vi "LINC Session Global.vi"(5 "target name":string, 6 "value in":i32, 7 "mode":T2, 8 "error in (no error)":errorcluster, 9 "reference in":refnum<vi>, 10 "listener in":refnum<k5>, 11 "connection in":refnum<k5>) -> (0 "error out":errorcluster, 1 "reference out":refnum<vi>[](array[refnum]), 2 "listener out":refnum<k5>[](array[refnum]), 3 "connections out":refnum<k5>[](array[refnum]), 4 "port config":T1[](array[typedef]))   [LabVIEW 2018, in "STEPkgDriver_LINC.lvlib"]
uses:
  STEPkgDriver_LINC.lvlib
  LINC Port Config.ctl
  LINC.lvclass
  LINC Global Session Mode.ctl
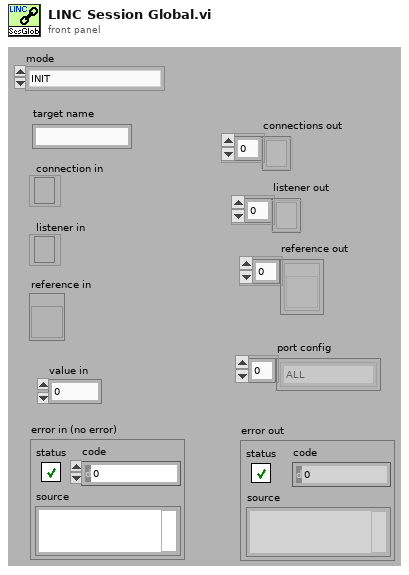
[diagram p1: front panel]
types:
  T1 = typedef "STEPkgDriver_LINC.lvlib/LINC Port Config.ctl" = enum16{"ALL", "CMD_ALL", "TLM_ALL", "TLM_BASIC"}
  T2 = typedef "STEPkgDriver_LINC.lvlib/LINC Global Session Mode.ctl" = enum16{"INIT", "CLEAR", "ADD_SESSION", "SET_CONNECTION", "SET_LISTENER", "SET_REFERENCE", "GET_SESSION"}
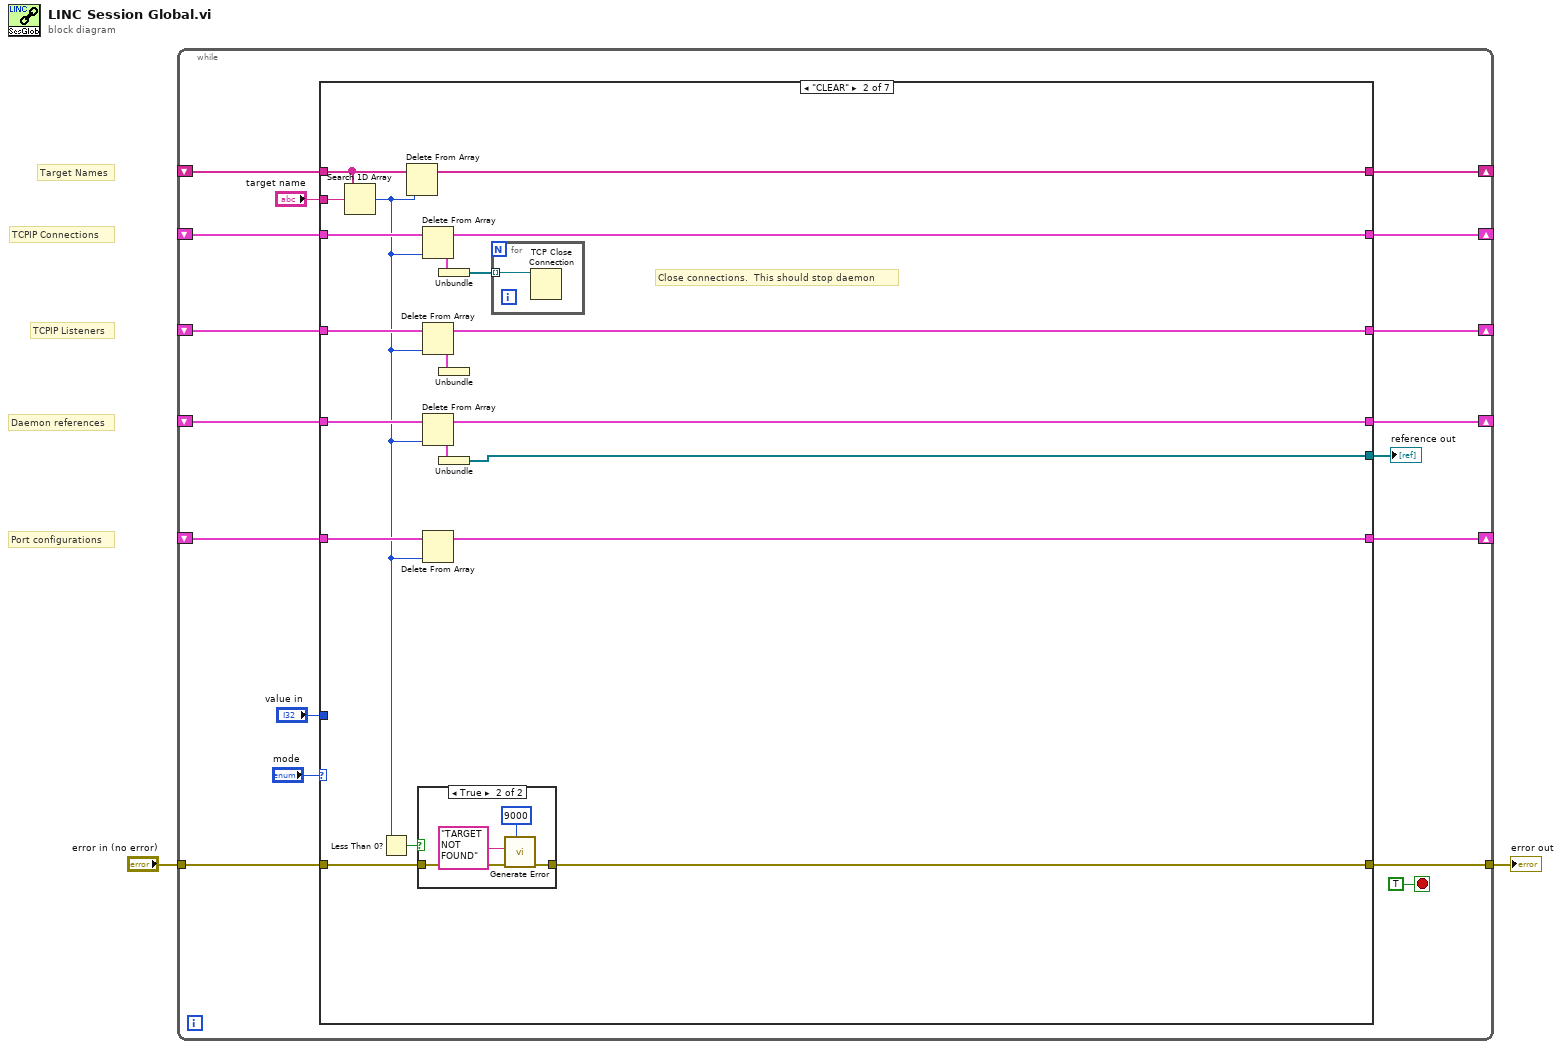
[diagram p0: block diagram]
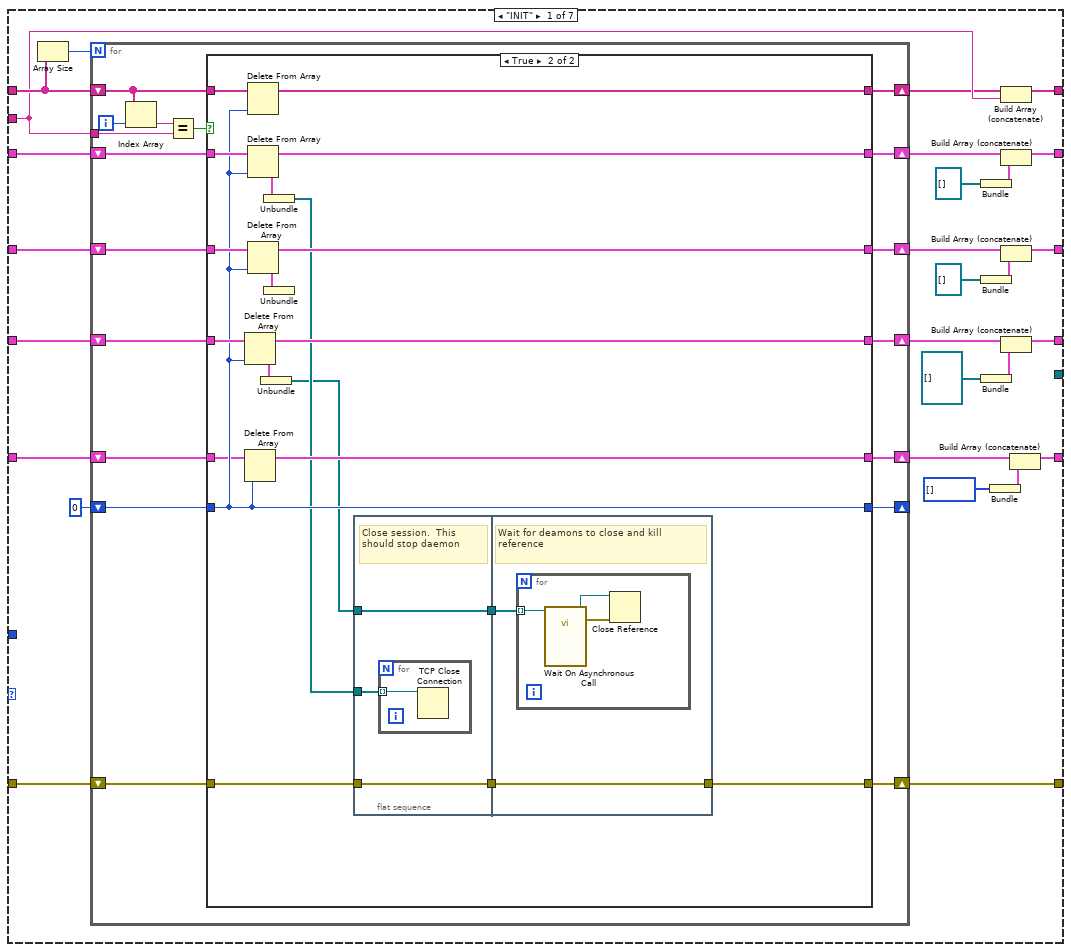
[diagram p2: hidden frame]
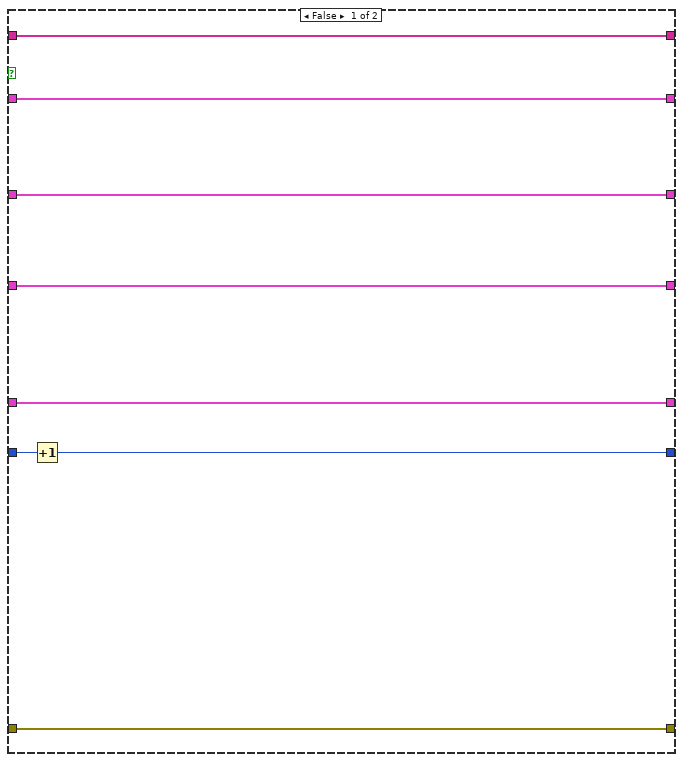
[diagram p3: hidden frame]
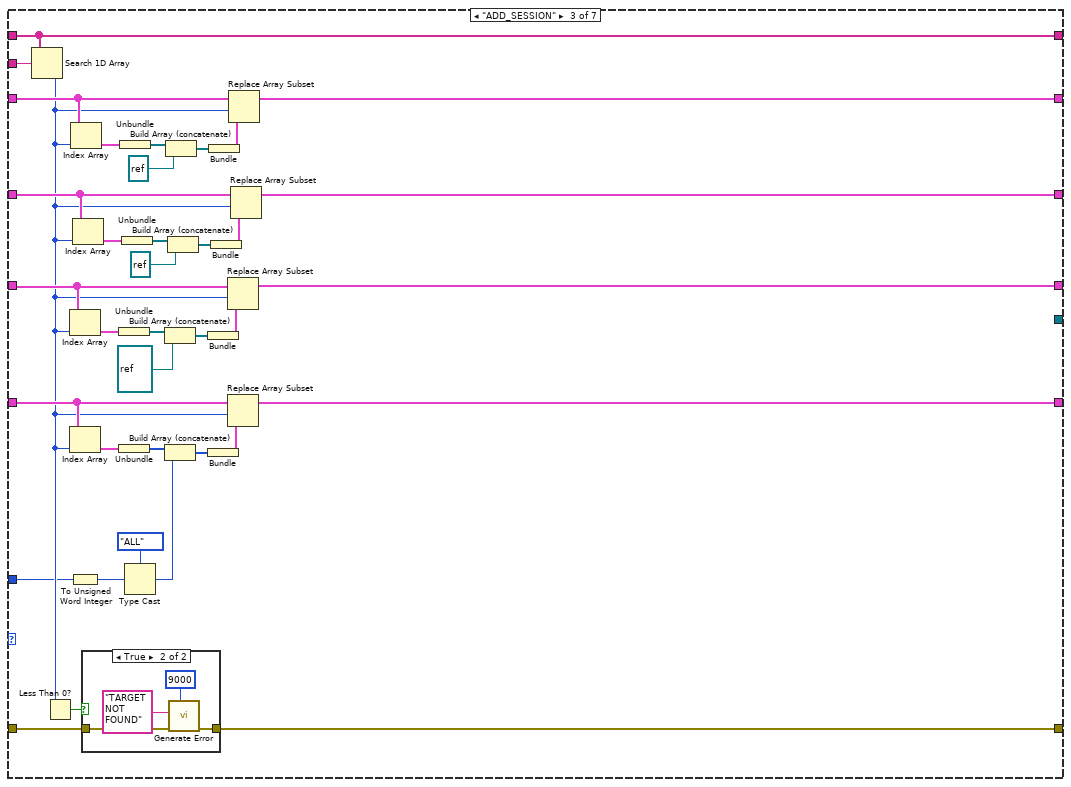
[diagram p5: hidden frame]
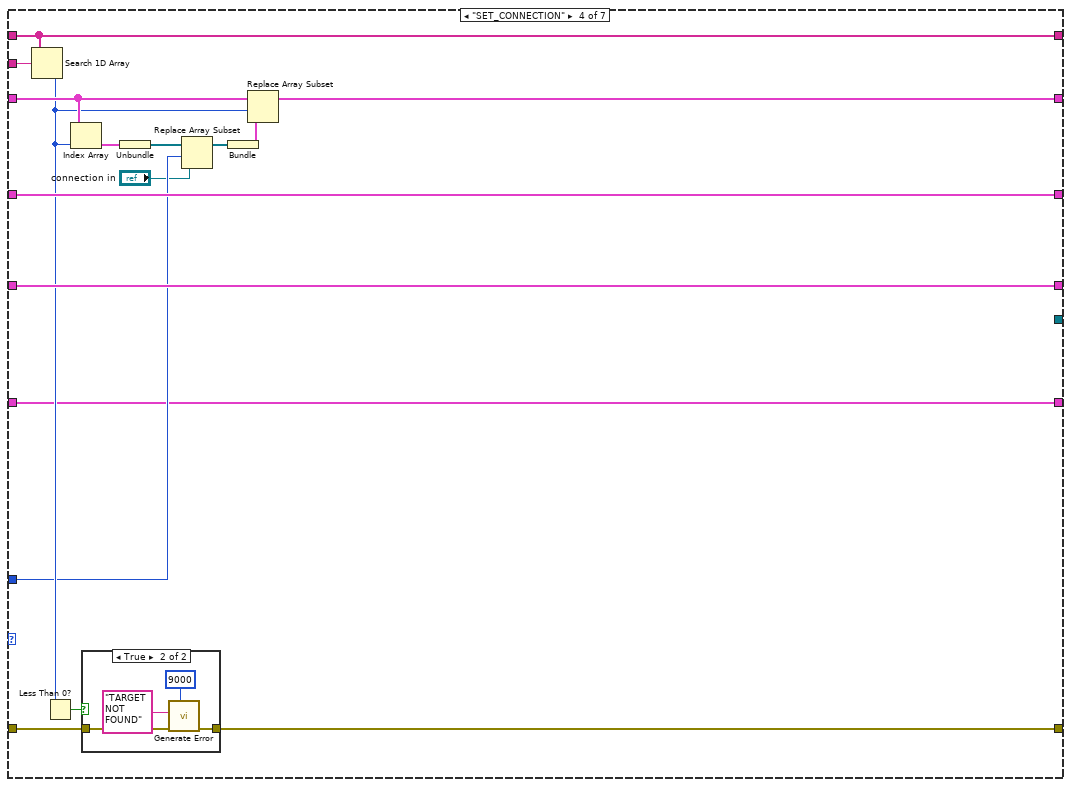
[diagram p7: hidden frame]
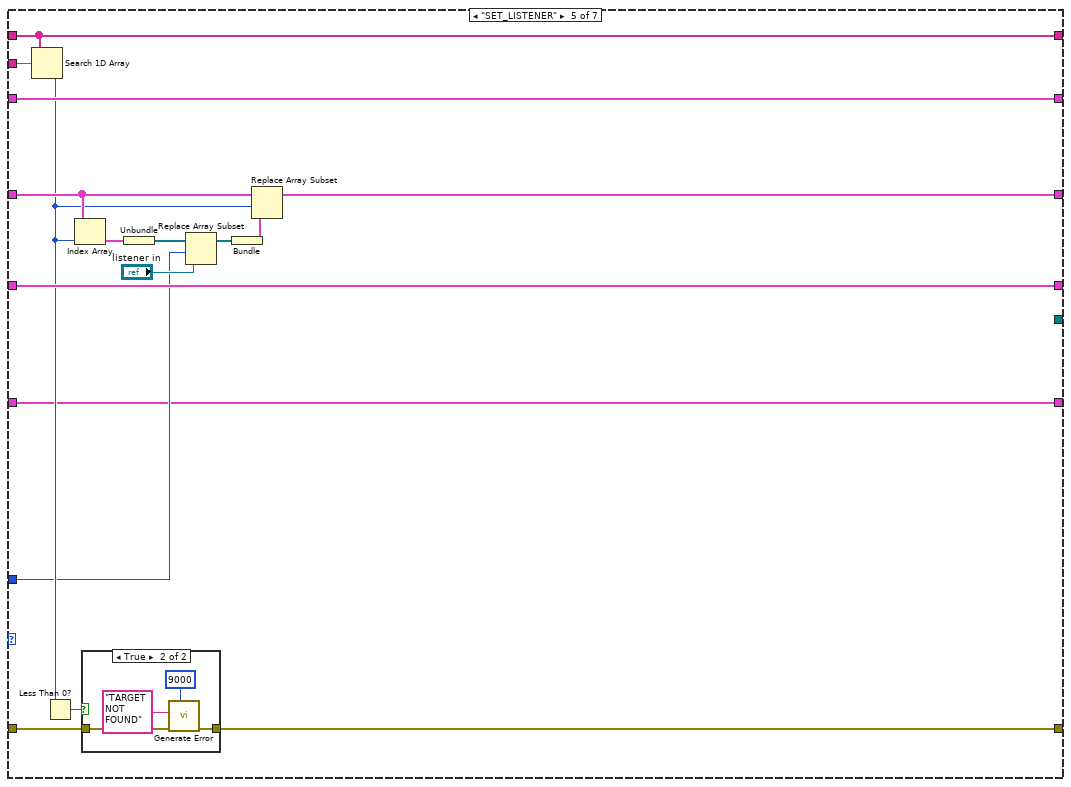
[diagram p9: hidden frame]
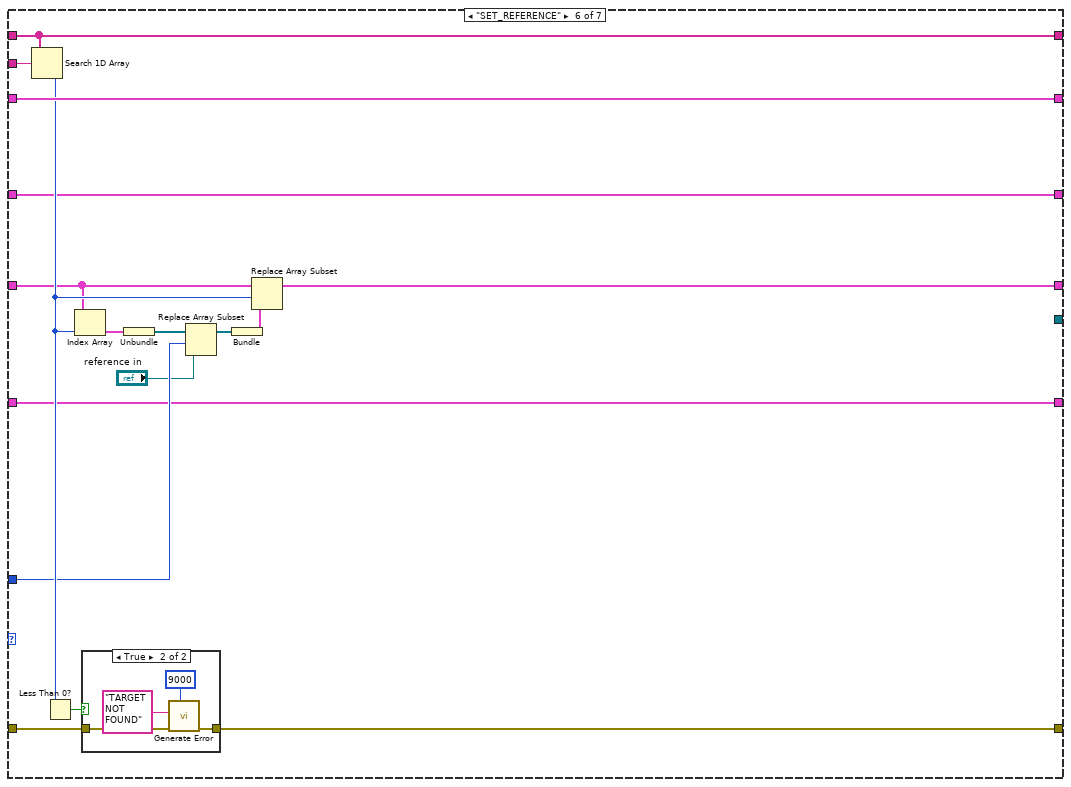
[diagram p11: hidden frame]
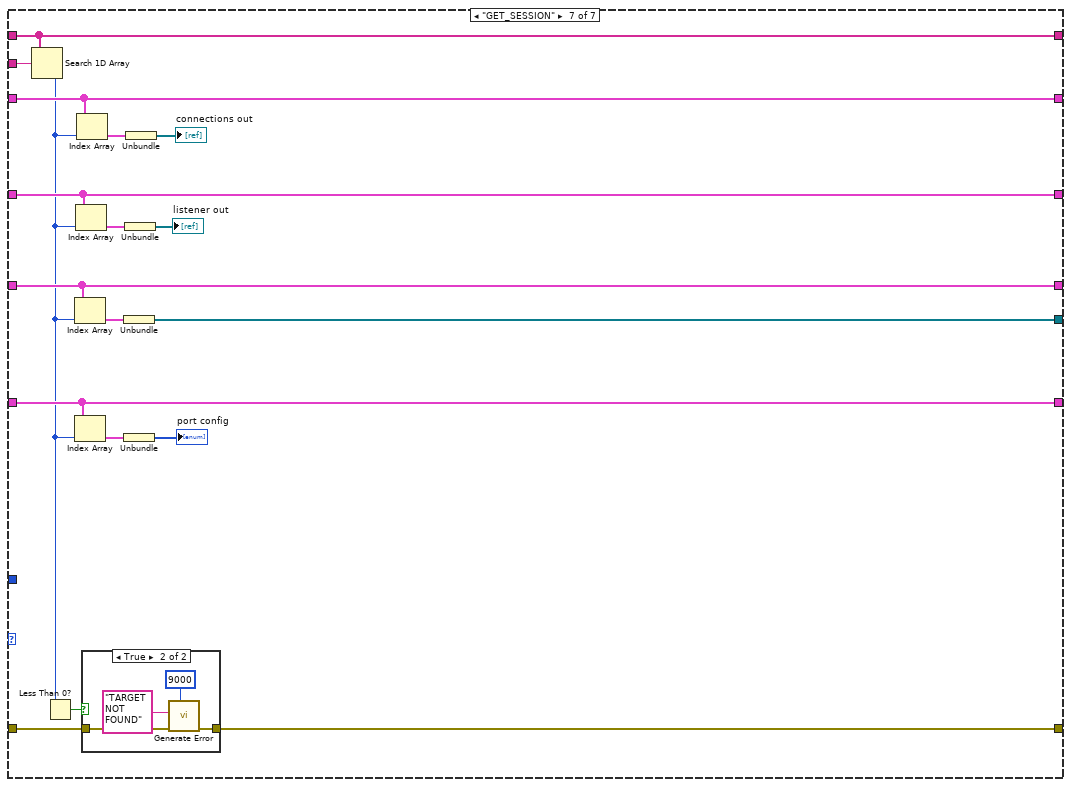
[diagram p13: hidden frame]
diagram:
  # "Target Names"
  # "Port configurations"
  # "Daemon references"
  # "TCPIP Listeners"
  # "TCPIP Connections"
  n1 = while {
    shift-right: [w17] -> _
    shift-left: _ -> [w18]
    tunnel: "error in (no error)" -> [w14]
    tunnel: [w13] -> w1
    shift-right: [w11] -> _
    shift-left: _ -> [w12]
    shift-right: [w9] -> _
    shift-left: _ -> [w10]
    shift-right: [w8] -> _
    shift-left: _ -> [w7]
    shift-right: [w4] -> _
    shift-left: _ -> [w5]
    stop <- TRUE stop-if-true
    n2 = case shown="\"CLEAR\"" "mode" {
      tunnel: w18 -> [w36 w121 w164 w186 w208 w230 w253]
      tunnel: [w47 w120 w164 w186 w208 w230 w253] -> w17
      tunnel: "target name" -> [w34 w122 w165 w187 w209 w231 w254]
      tunnel: w14 -> [w21 w118 w160 w183 w205 w227 w251]
      tunnel: [w20 w104 w161 w182 w204 w226 w250] -> w13
      tunnel: w12 -> [w33 w117 w159 w178 w207 w229 w249]
      tunnel: [w46 w116 w163 w177 w207 w229 w249] -> w11
      tunnel: w10 -> [w30 w115 w148 w185 w198 w218 w245]
      tunnel: [w41 w114 w147 w185 w197 w218 w245] -> w9
      tunnel: w7 -> [w29 w113 w142 w181 w203 w219 w244]
      tunnel: [w40 w112 w141 w181 w203 w217 w244] -> w8
      tunnel: "value in" -> [_ _ w133 w173 w194 w220 _]
      tunnel: w5 -> [w25 w108 w136 w171 w193 w216 w240]
      tunnel: [w23 w107 w135 w171 w193 w216 w240] -> w4
      tunnel: [_ w103 _ _ _ _ w237] -> w3
      frame "INIT" {
        w26 = T1[] [] items=["ALL", "CMD_ALL", "TLM_ALL", "TLM_BASIC"]
        n3 = Array Size(array=w36) -> (size(s)=w35:i32)
        n4 = for {
          N: w35 -> [_]
          shift-right: [w58] -> w32
          shift-left: w36 -> [w64]
          shift-right: [w57] -> w31
          shift-left: w33 -> [w63]
          shift-right: [w56] -> w28
          shift-left: w30 -> [w62]
          tunnel: w34 -> [w60]
          shift-right: [w54] -> _
          shift-left: 0 -> [w55]
          shift-right: [w53] -> w27
          shift-left: w29 -> [w52]
          shift-right: [w50] -> w24
          shift-left: w25 -> [w51]
          shift-right: [w48] -> w20
          shift-left: w21 -> [w49]
          i -> [w65]
          n5 = Index Array(array=w64, index=w65) -> (element=w61:string)
          n6 = Equal?(x=w61, y=w60) -> (x = y?=w59:bool)
          n7 = case shown="True" w59 {
            tunnel: w64 -> [w73 w93]
            tunnel: w63 -> [w72 w91]
            tunnel: w62 -> [w71 w90]
            tunnel: [w73 w92] -> w58
            tunnel: [w72 w89] -> w57
            tunnel: [w71 w88] -> w56
            tunnel: w55 -> [w70 w82]
            tunnel: [w69 w82] -> w54
            tunnel: w52 -> [w68 w86]
            tunnel: [w68 w87] -> w53
            tunnel: w51 -> [w67 w81]
            tunnel: [w67 w80] -> w50
            tunnel: w49 -> [w66 w79]
            tunnel: [w66 w78] -> w48
            frame False {
              n8 = Increment(x=w70) -> (x+1=w69:i32)
            }
            frame True {
              n9 = Delete From Array(array=w86, index=w82) -> (deleted portion=w83:cluster{refnum<vi>[]}, array with subset deleted=w87:cluster{refnum<vi>[]}[])  [unwired: 1 in]
              n10 = Delete From Array(array=w81, index=w82) -> (array with subset deleted=w80:cluster{T1[]}[])  [unwired: 1 in, 1 out]
              n11 = Delete From Array(array=w93, index=w82) -> (array with subset deleted=w92:string[])  [unwired: 1 in, 1 out]
              n12 = Delete From Array(array=w91, index=w82) -> (deleted portion=w85:cluster{refnum<k5>[]}, array with subset deleted=w89:cluster{refnum<k5>[]}[])  [unwired: 1 in]
              n13 = Delete From Array(array=w90, index=w82) -> (deleted portion=w84:cluster{refnum<k5>[]}, array with subset deleted=w88:cluster{refnum<k5>[]}[])  [unwired: 1 in]
              n14 = Unbundle(w83) -> (w76:refnum<vi>[])
              n15 = Unbundle(w85) -> (w77:refnum<k5>[])
              n16 = Unbundle(w84) -> ()  [unwired: 1 out]
              n17 = flat-sequence {
                tunnel: w79 -> [w96]
                tunnel: [w96] -> w75
                tunnel: w77 -> [w95]
                tunnel: [w94] -> w74
                tunnel: w76 -> [w94]
                tunnel: w75 -> [w98]
                tunnel: w74 -> [w99]
                tunnel: [w98] -> w78
                frame #0 {
                  # "Close session.  This should stop daemon"
                  n18 = for {
                    tunnel: w95 -> [w97] mode=indexing
                    n19 = TCP Close Connection(connection ID=w97) -> ()  [unwired: 2 in, 2 out]
                  }
                }
                frame #1 {
                  # "Wait for deamons to close and kill reference"
                  n20 = for {
                    tunnel: w99 -> [w102] mode=indexing
                    n21 = call-by-ref "Wait On Asynchronous Call"(reference=w102) -> (reference out=w100:refnum<vi>, error out=w101:errorcluster)  [unwired: 13 in]
                    n22 = Close Reference(reference=w100, error in (no error)=w101) -> ()  [unwired: 1 out]
                  }
                }
              }
            }
          }
        }
        n23 = Bundle(refnum<k5>[] []) -> (w44:cluster{refnum<k5>[]})  [unwired: 1 in]
        n24 = Bundle(refnum<k5>[] []) -> (w43:cluster{refnum<k5>[]})  [unwired: 1 in]
        n25 = Bundle(refnum<vi>[] []) -> (w38:cluster{refnum<vi>[]})  [unwired: 1 in]
        n26 = Bundle(w26) -> (w22:cluster{T1[]})  [unwired: 1 in]
        n27 = Build Array (concatenate)(w32, w34) -> (w47:string[])
        n28 = Build Array (concatenate)(w31, w44) -> (w46:cluster{refnum<k5>[]}[])
        n29 = Build Array (concatenate)(w28, w43) -> (w41:cluster{refnum<k5>[]}[])
        n30 = Build Array (concatenate)(w27, w38) -> (w40:cluster{refnum<vi>[]}[])
        n31 = Build Array (concatenate)(w24, w22) -> (w23:cluster{T1[]}[])
      }
      frame "CLEAR" {
        # "Close connections.  This should stop daemon"
        n32 = Search 1D Array(1D array=w121, element=w122) -> (index of element=w106:i32)  [unwired: 1 in]
        n33 = Less Than 0?(x=w106) -> (x < 0?=w119:bool)
        n34 = Delete From Array(array=w121, index=w106) -> (array with subset deleted=w120:string[])  [unwired: 1 in, 1 out]
        n35 = case shown="True" w119 {
          tunnel: w118 -> [w124 w128]
          tunnel: [w124 w127] -> w104
          frame False {
          }
          frame True {
            n36 = call "Generate Error.vi"("error code (-1301)"=9000, "error in"=w128, "description"="TARGET NOT FOUND") -> ("error out"=w127:errorcluster)  [unwired: 8 in]
          }
        }
        n37 = Delete From Array(array=w117, index=w106) -> (deleted portion=w111:cluster{refnum<k5>[]}, array with subset deleted=w116:cluster{refnum<k5>[]}[])  [unwired: 1 in]
        n38 = Delete From Array(array=w115, index=w106) -> (deleted portion=w110:cluster{refnum<k5>[]}, array with subset deleted=w114:cluster{refnum<k5>[]}[])  [unwired: 1 in]
        n39 = Delete From Array(array=w113, index=w106) -> (deleted portion=w109:cluster{refnum<vi>[]}, array with subset deleted=w112:cluster{refnum<vi>[]}[])  [unwired: 1 in]
        n40 = Delete From Array(array=w108, index=w106) -> (array with subset deleted=w107:cluster{T1[]}[])  [unwired: 1 in, 1 out]
        n41 = Unbundle(w111) -> (w105:refnum<k5>[])
        n42 = Unbundle(w110) -> ()  [unwired: 1 out]
        n43 = Unbundle(w109) -> (w103:refnum<vi>[])
        n44 = for {
          tunnel: w105 -> [w123] mode=indexing
          n45 = TCP Close Connection(connection ID=w123) -> ()  [unwired: 2 in, 2 out]
        }
      }
      frame "ADD_SESSION" {
        n46 = Search 1D Array(1D array=w164, element=w165) -> (index of element=w134:i32)  [unwired: 1 in]
        n47 = Less Than 0?(x=w134) -> (x < 0?=w162:bool)
        n48 = Index Array(array=w142, index=w134) -> (element=w146:cluster{refnum<vi>[]})
        n49 = Index Array(array=w136, index=w134) -> (element=w137:cluster{T1[]})
        n50 = To Unsigned Word Integer(number=w133) -> (unsigned 16bit integer=w130:u16)
        n51 = Index Array(array=w159, index=w134) -> (element=w158:cluster{refnum<k5>[]})
        n52 = Index Array(array=w148, index=w134) -> (element=w149:cluster{refnum<k5>[]})
        n53 = case shown="True" w162 {
          tunnel: w160 -> [w166 w170]
          tunnel: [w166 w169] -> w161
          frame False {
          }
          frame True {
            n54 = call "Generate Error.vi"("error code (-1301)"=9000, "error in"=w170, "description"="TARGET NOT FOUND") -> ("error out"=w169:errorcluster)  [unwired: 8 in]
          }
        }
        n55 = Unbundle(w146) -> (w145:refnum<vi>[])
        n56 = Unbundle(w137) -> (w138:T1[])
        n57 = Unbundle(w158) -> (w157:refnum<k5>[])
        n58 = Unbundle(w149) -> (w150:refnum<k5>[])
        n59 = Type Cast(type=LINC_Port_Config."ALL" ("port config"), x=w130) -> (*(type *) &x=w131:T1)
        n60 = Build Array (concatenate)(w145, refnum<vi> refnum) -> (w144:refnum<vi>[])
        n61 = Build Array (concatenate)(w138, w131) -> (w139:T1[])
        n62 = Build Array (concatenate)(w157, refnum<k5> refnum ("connection in")) -> (w155:refnum<k5>[])
        n63 = Build Array (concatenate)(w150, refnum<k5> refnum ("connection in")) -> (w152:refnum<k5>[])
        n64 = Bundle(w144) -> (w143:cluster{refnum<vi>[]})  [unwired: 1 in]
        n65 = Bundle(w139) -> (w140:cluster{T1[]})  [unwired: 1 in]
        n66 = Bundle(w155) -> (w154:cluster{refnum<k5>[]})  [unwired: 1 in]
        n67 = Bundle(w152) -> (w153:cluster{refnum<k5>[]})  [unwired: 1 in]
        n68 = Replace Array Subset(array=w142, new element=w143, index=w134) -> (w141:cluster{refnum<vi>[]}[])
        n69 = Replace Array Subset(array=w136, new element=w140, index=w134) -> (w135:cluster{T1[]}[])
        n70 = Replace Array Subset(array=w159, new element=w154, index=w134) -> (w163:cluster{refnum<k5>[]}[])
        n71 = Replace Array Subset(array=w148, new element=w153, index=w134) -> (w147:cluster{refnum<k5>[]}[])
      }
      frame "SET_CONNECTION" {
        n72 = Search 1D Array(1D array=w186, element=w187) -> (index of element=w176:i32)  [unwired: 1 in]
        n73 = Less Than 0?(x=w176) -> (x < 0?=w184:bool)
        n74 = Index Array(array=w178, index=w176) -> (element=w180:cluster{refnum<k5>[]})
        n75 = case shown="True" w184 {
          tunnel: w183 -> [w188 w192]
          tunnel: [w188 w191] -> w182
          frame False {
          }
          frame True {
            n76 = call "Generate Error.vi"("error code (-1301)"=9000, "error in"=w192, "description"="TARGET NOT FOUND") -> ("error out"=w191:errorcluster)  [unwired: 8 in]
          }
        }
        n77 = Unbundle(w180) -> (w175:refnum<k5>[])
        n78 = Replace Array Subset(array=w175, new element="connection in", index=w173) -> (w174:refnum<k5>[])
        n79 = Bundle(w174) -> (w179:cluster{refnum<k5>[]})  [unwired: 1 in]
        n80 = Replace Array Subset(array=w178, new element=w179, index=w176) -> (w177:cluster{refnum<k5>[]}[])
      }
      frame "SET_LISTENER" {
        n81 = Search 1D Array(1D array=w208, element=w209) -> (index of element=w196:i32)  [unwired: 1 in]
        n82 = Less Than 0?(x=w196) -> (x < 0?=w206:bool)
        n83 = Index Array(array=w198, index=w196) -> (element=w202:cluster{refnum<k5>[]})
        n84 = case shown="True" w206 {
          tunnel: w205 -> [w210 w214]
          tunnel: [w210 w213] -> w204
          frame False {
          }
          frame True {
            n85 = call "Generate Error.vi"("error code (-1301)"=9000, "error in"=w214, "description"="TARGET NOT FOUND") -> ("error out"=w213:errorcluster)  [unwired: 8 in]
          }
        }
        n86 = Unbundle(w202) -> (w200:refnum<k5>[])
        n87 = Replace Array Subset(array=w200, new element="listener in", index=w194) -> (w199:refnum<k5>[])
        n88 = Bundle(w199) -> (w201:cluster{refnum<k5>[]})  [unwired: 1 in]
        n89 = Replace Array Subset(array=w198, new element=w201, index=w196) -> (w197:cluster{refnum<k5>[]}[])
      }
      frame "SET_REFERENCE" {
        n90 = Search 1D Array(1D array=w230, element=w231) -> (index of element=w221:i32)  [unwired: 1 in]
        n91 = Less Than 0?(x=w221) -> (x < 0?=w228:bool)
        n92 = Index Array(array=w219, index=w221) -> (element=w225:cluster{refnum<vi>[]})
        n93 = case shown="True" w228 {
          tunnel: w227 -> [w232 w236]
          tunnel: [w232 w235] -> w226
          frame False {
          }
          frame True {
            n94 = call "Generate Error.vi"("error code (-1301)"=9000, "error in"=w236, "description"="TARGET NOT FOUND") -> ("error out"=w235:errorcluster)  [unwired: 8 in]
          }
        }
        n95 = Unbundle(w225) -> (w223:refnum<vi>[])
        n96 = Replace Array Subset(array=w223, new element="reference in", index=w220) -> (w222:refnum<vi>[])
        n97 = Bundle(w222) -> (w224:cluster{refnum<vi>[]})  [unwired: 1 in]
        n98 = Replace Array Subset(array=w219, new element=w224, index=w221) -> (w217:cluster{refnum<vi>[]}[])
      }
      frame "GET_SESSION" {
        n99 = Search 1D Array(1D array=w253, element=w254) -> (index of element=w239:i32)  [unwired: 1 in]
        n100 = Less Than 0?(x=w239) -> (x < 0?=w252:bool)
        n101 = Index Array(array=w244, index=w239) -> (element=w246:cluster{refnum<vi>[]})
        n102 = Index Array(array=w240, index=w239) -> (element=w241:cluster{T1[]})
        n103 = Index Array(array=w245, index=w239) -> (element=w247:cluster{refnum<k5>[]})
        n104 = Index Array(array=w249, index=w239) -> (element=w248:cluster{refnum<k5>[]})
        n105 = case shown="True" w252 {
          tunnel: w251 -> [w255 w259]
          tunnel: [w255 w258] -> w250
          frame False {
          }
          frame True {
            n106 = call "Generate Error.vi"("error code (-1301)"=9000, "error in"=w259, "description"="TARGET NOT FOUND") -> ("error out"=w258:errorcluster)  [unwired: 8 in]
          }
        }
        n107 = Unbundle(w246) -> (w237:refnum<vi>[])
        n108 = Unbundle(w241) -> (→"port config":T1[])
        n109 = Unbundle(w247) -> (→"listener out":refnum<k5>[])
        n110 = Unbundle(w248) -> (→"connections out":refnum<k5>[])
      }
    }
    "reference out" <- w3
  }
  "error out" <- w1
